vi "Process.vi"(8 "error in (no error)":errorcluster, 9 "Panel":refnum<class "Panel Controller Interface.lvclass">, 10 "Console Reply.lvclass":refnum<class "Console Reply.lvclass">, 11 "Panel Behavior.lvclass":refnum<class "Panel Behavior.lvclass">) -> (0 "error out":errorcluster, 3 "Panel Behavior.lvclass":refnum<class "Panel Behavior.lvclass">)   [LabVIEW 2015, in "EditPanel API.lvlib" / "Panel Behavior.lvclass"]
uses:
  Panel Behavior.lvclass
  Console Reply/Console Reply/Console Reply.lvclass
  Panel Control_Interface/Panel_interface/Panel Controller Interface.lvclass
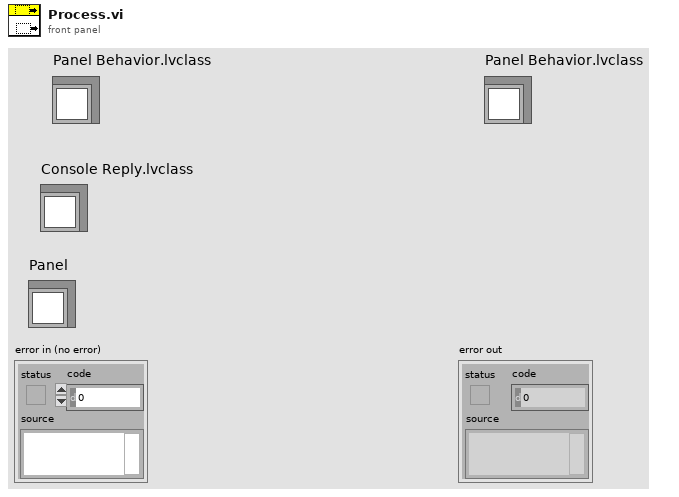
[diagram p1: front panel]
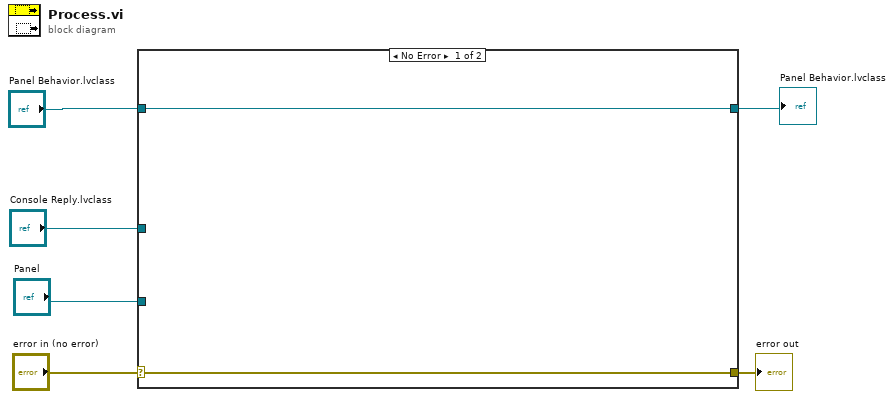
[diagram p0: block diagram]
diagram:
  n1 = case shown="No Error" "error in (no error)" {
    selector: "error in (no error)" -> [w7 w10]
    tunnel: [w7 w10] -> w5
    tunnel: [w8 w9] -> w3
    tunnel: "Panel Behavior.lvclass" -> [w8 w9]
    tunnel: "Console Reply.lvclass" -> [_ _]
    tunnel: "Panel" -> [_ _]
    frame No Error {
    }
    frame Error {
    }
  }
  "error out" <- w5
  "Panel Behavior.lvclass" <- w3
